vi "Insert Right SubPanel.vi"(8 "error in (no error)":errorcluster, 9 "ActorQName":string, 10 "ActorVI Ref":refnum<vi>, 11 "UI_Left_Right in":refnum<class "UI_Left_Right.lvclass">) -> (0 "error out":errorcluster, 3 "UI_Left_Right out":refnum<class "UI_Left_Right.lvclass">)   [LabVIEW 2021, in "UI_Left_Right.lvclass"]
uses:
  UI_Left_Right.lvclass
  C:/Program Files (x86)/National Instruments/LabVIEW 2021/vi.lib/ActorFramework/Actor/Actor.lvclass
  UI_Left_Right.lvclass/UI_Left_Right.ctl
  <vilib>/ActorFramework/Actor/Actor.lvclass/Actor.ctl
  <vilib>/ActorFramework/Message Enqueuer/Message Enqueuer.lvclass/Message Enqueuer.ctl
  <vilib>/ActorFramework/Message Enqueuer/Enqueue.vi
  <userlib>/John_Lib/AbstractActorTemplate/UIActorTop Messages/UI Initialize Msg/UI Initialize Msg.lvclass
  C:/Program Files (x86)/National Instruments/LabVIEW 2021/vi.lib/ActorFramework/Message/Message.lvclass
  <vilib>/ActorFramework/Message Priority Queue/Priority Enqueue.vi
  <vilib>/ActorFramework/Actor/Actor.lvclass
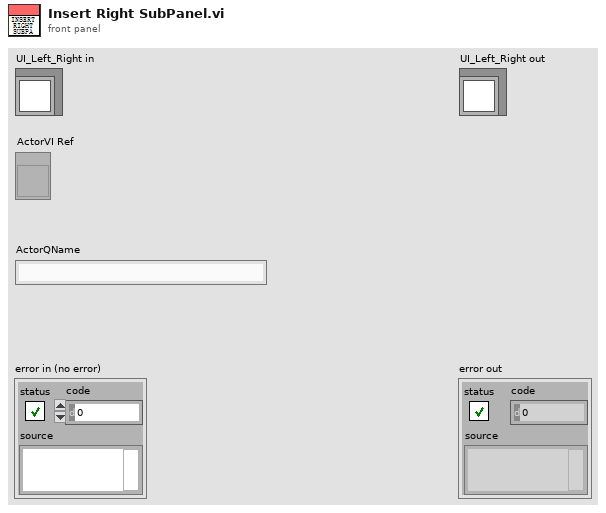
[diagram p1: front panel]
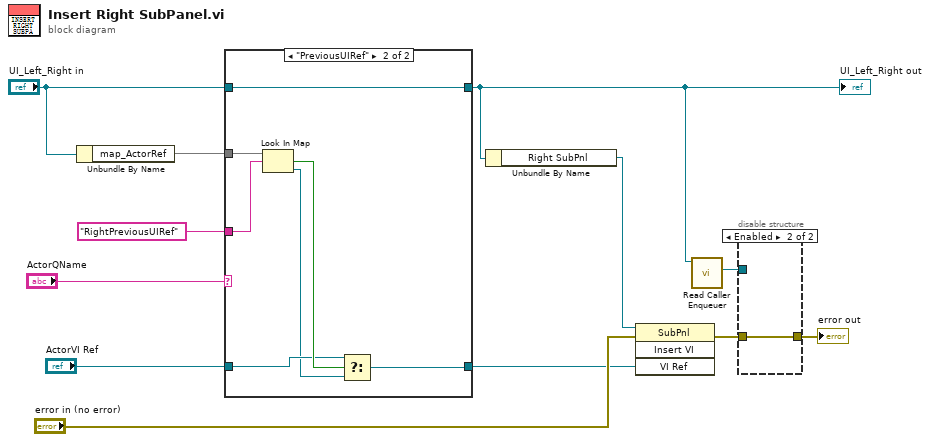
[diagram p0: block diagram]
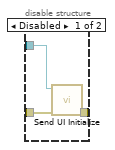
[diagram p2: hidden frame]
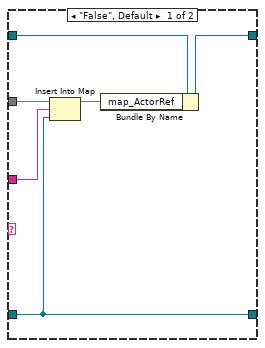
[diagram p3: hidden frame]
diagram:
  n1 = Unbundle By Name("UI_Left_Right in") -> ("map_ActorRef"=w6:map{string, refnum<vi>})
  n2 = case shown="\"PreviousUIRef\"" "ActorQName" {
    tunnel: [w17 w25] -> w2
    tunnel: "UI_Left_Right in" -> [w18 w25]
    tunnel: w6 -> [w16 w24]
    tunnel: "RightPreviousUIRef" ("key") -> [w14 w23]
    tunnel: "ActorVI Ref" -> [w13 w21]
    tunnel: [w13 w19] -> w3
    frame "False", Default {
      n3 = Insert Into Map(map in=w16, key=w14, value=w13) -> (map out=w15:map{string, refnum<vi>})  [unwired: 2 out]
      n4 = Bundle By Name(cluster=w18, "map_ActorRef"=w15) -> (w17:refnum<class "UI_Left_Right.lvclass">)
    }
    frame "PreviousUIRef" {
      n5 = Look In Map(map=w24, key=w23) -> (key not found?=w22:bool, value=w20:refnum<vi>)  [unwired: 1 in]
      n6 = Select(t=w21, s=w22, f=w20) -> (s? t:f=w19:refnum<vi>)
    }
  }
  "UI_Left_Right out" <- w2
  n7 = Unbundle By Name(w2) -> ("Right SubPnl"=w1:refnum<vi>)
  n8 = invoke class="SubPnl" method="Insert VI"(reference=w1, error in="error in (no error)", "VI Ref"=w3) -> (error out=w10:errorcluster)  [unwired: 1 in, 3 out]
  n9 = call <vilib>:"Read Caller Enqueuer.vi"("Actor"=w2) -> ("Caller Enqueuer"=w11:refnum<class "Message Enqueuer.lvclass">)  [unwired: 10 in]
  n10 = disable-structure shown="Enabled" {
    disable-tunnel: w11 -> [w28 _]
    disable-tunnel: w10 -> [w27 w29]
    disable-tunnel: [w26 w29] -> w9
    frame Disabled {
      n11 = call <userlib>:"Send UI Initialize.vi"("error in (no error)"=w27, "Message Enqueuer"=w28) -> ("error out"=w26:errorcluster)  [unwired: 8 in, 1 out]
    }
    frame Enabled {
    }
  }
  "error out" <- w9
